vi "Utility - Bytes to Values.vi"(10 "DataBuffer":u8[](array[numeric]) format="%.0x") -> (1 "Period":u32, 2 "Measurement Value":sgl)   [LabVIEW 2018]
panel:
  # "The VI is just a utility used to convert\nraw data from the meter's buffer into\nmeasurement values.  This utility is\nused inside some of the other VIs\nincluded here."
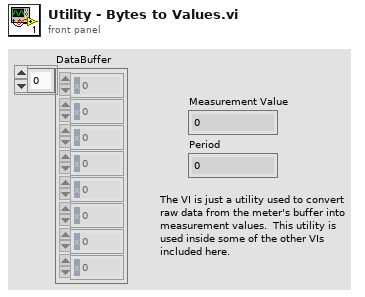
[diagram p1: front panel]
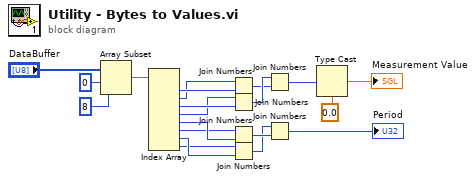
[diagram p0: block diagram]
diagram:
  n1 = Array Subset(array="DataBuffer", index=0, length=8) -> (w12:u8[])
  n2 = Index Array(array=w12) -> (element #1=w13:u8, element #2=w11:u8, element #3=w10:u8, element #4=w9:u8, element #5=w8:u8, element #6=w7:u8, element #7=w6:u8, element #8=w5:u8)  [unwired: 8 in]
  n3 = Join Numbers(hi=w11, lo=w13) -> ((hi.lo)=w16:u16)
  n4 = Join Numbers(hi=w9, lo=w10) -> ((hi.lo)=w17:u16)
  n5 = Join Numbers(hi=w7, lo=w8) -> ((hi.lo)=w15:u16)
  n6 = Join Numbers(hi=w5, lo=w6) -> ((hi.lo)=w14:u16)
  n7 = Join Numbers(hi=w17, lo=w16) -> ((hi.lo)=w3:u32)
  n8 = Join Numbers(hi=w14, lo=w15) -> ((hi.lo)=→"Period":u32)
  n9 = Type Cast(type=sgl 0.0, x=w3) -> (*(type *) &x=→"Measurement Value":sgl)
